vi "ENBW RC.vi"(10 "time constant (s)":dbl, 11 "filter order":i32) -> (3 "ENBW (Hz)":dbl)   [LabVIEW 2019, in "DSP.lvclass"]
uses:
  DSP.lvclass
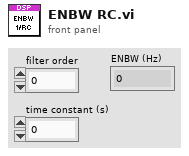
[diagram p1: front panel]
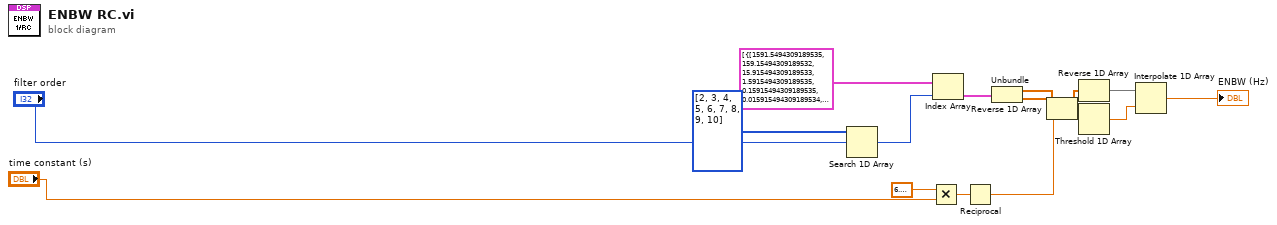
[diagram p0: block diagram]
diagram:
  n1 = Search 1D Array(1D array=i32[] [2, 3, 4, 5, 6, 7, 8, 9, 10] ("Array"), element="filter order") -> (index of element=w4:i32)  [unwired: 1 in]
  n2 = Multiply(x=6.283185307179586, y="time constant (s)") -> (x*y=w7:dbl)
  n3 = Index Array(array=cluster{dbl[], dbl[]}[] [{[1591.5494309189535, 159.15494309189532, 15.915494309189533, 1.5915494309189535, 0.15915494309189535, 0.015915494309189534, 0.0015915494309189533], [495.20998273974345, 62.4229271880735, 6.248240956900394, 0.6239944736705205, 0.06151755931078814, 0.005411201053636981, 0.005411201053636981]}, {[1591.5494309189535, 159.15494309189532, 15.915494309189533, 1.5915494309189535, 0.15915494309189535, 0.015915494309189534, 0.0015915494309189533], [371.3956776627174, 46.81692220466569, 4.685930770818215, 0.46774661763014, 0.04589562814034717, 0.0038711399018682845, 0.0038711399018682845]}, {[1591.5494309189535, 159.15494309189532, 15.915494309189533, 1.5915494309189535, 0.15915494309189535, 0.015915494309189534, 0.0015915494309189533], [309.49430057164426, 39.01393130880754, 3.9047756840751426, 0.38962263434350103, 0.03808423602056431, 0.003096524200890878, 0.003096524200890878]}, {[1591.5494309189535, 159.15494309189532, 15.915494309189533, 1.5915494309189535, 0.15915494309189535, 0.015915494309189534, 0.0015915494309189533], [270.8066641476653, 34.137063450841815, 3.4165537778564654, 0.3407953602555583, 0.03320410909560028, 0.0026273275317945832, 0.0026273275317945832]}, {[1591.5494309189535, 159.15494309189532, 15.915494309189533, 1.5915494309189535, 0.15915494309189535, 0.015915494309189534, 0.0015915494309189533], [243.72553582713797, 30.723256384408266, 3.0747984352453623, 0.3066161794363722, 0.029787236245632936, 0.002292347323821602, 0.002292347323821602]}, {[1591.5494309189535, 159.15494309189532, 15.915494309189533, 1.5915494309189535, 0.15915494309189535, 0.015915494309189534, 0.0015915494309189533], [223.41478006854084, 28.162901267388566, 2.818481944562892, 0.280981955447431, 0.027226067256090846, 0.002051657977834849, 0.002051657977834849]}, {[1591.5494309189535, 159.15494309189532, 15.915494309189533, 1.5915494309189535, 0.15915494309189535, 0.015915494309189534, 0.0015915494309189533], [207.4563743543134, 26.151193765188, 2.617090407395517, 0.2608406885772801, 0.02521290661445163, 0.0018563064603065826, 0.0018563064603065826]}, {[1591.5494309189535, 159.15494309189532, 15.915494309189533, 1.5915494309189535, 0.15915494309189535, 0.015915494309189534, 0.0015915494309189533], [194.49019515799765, 24.516681471943965, 2.4534597968174388, 0.24447604364472594, 0.023578442690996026, 0.0017059341570062516, 0.0017059341570062516]}, {[1591.5494309189535, 159.15494309189532, 15.915494309189533, 1.5915494309189535, 0.15915494309189535, 0.015915494309189534, 0.0015915494309189533], [183.68506137802152, 23.15458792453259, 2.3171009461712795, 0.23083875181365865, 0.02221560141426528, 0.00157492466432026, 0.00157492466432026]}] ("XY Graph 6"), index=w4) -> (element=w8:cluster{dbl[], dbl[]})
  n4 = Reciprocal(x=w7) -> (1/x=w10:dbl)
  n5 = Unbundle(w8) -> (w9:dbl[], w11:dbl[])
  n6 = Reverse 1D Array(array=w9) -> (reversed array=w14:dbl[])
  n7 = Reverse 1D Array(array=w11) -> (reversed array=w15:dbl[])
  n8 = Threshold 1D Array(2:w10, 3:w14) -> (0:w12:dbl)  [unwired: 1 in]
  n9 = Interpolate 1D Array(1:w12, 2:w15) -> (0:→"ENBW (Hz)":dbl)
